vi "Build Project Directory Menu.vi"(9 "Coords":T1, 10 "Project Tree Menu":refnum<k9>, 11 "Project Tree":refnum<vi>) -> (3 "Discard":bool)   [LabVIEW 2015, in "Editor.lvclass"]
uses:
  Editor.lvclass
  <vilib>/Utility/miscctls.llb/LVPoint32TypeDef.ctl
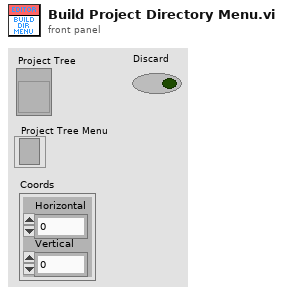
[diagram p1: front panel]
types:
  T1 = typedef "LVPoint32TypeDef.ctl" = cluster{"Horizontal":i32, "Vertical":i32}
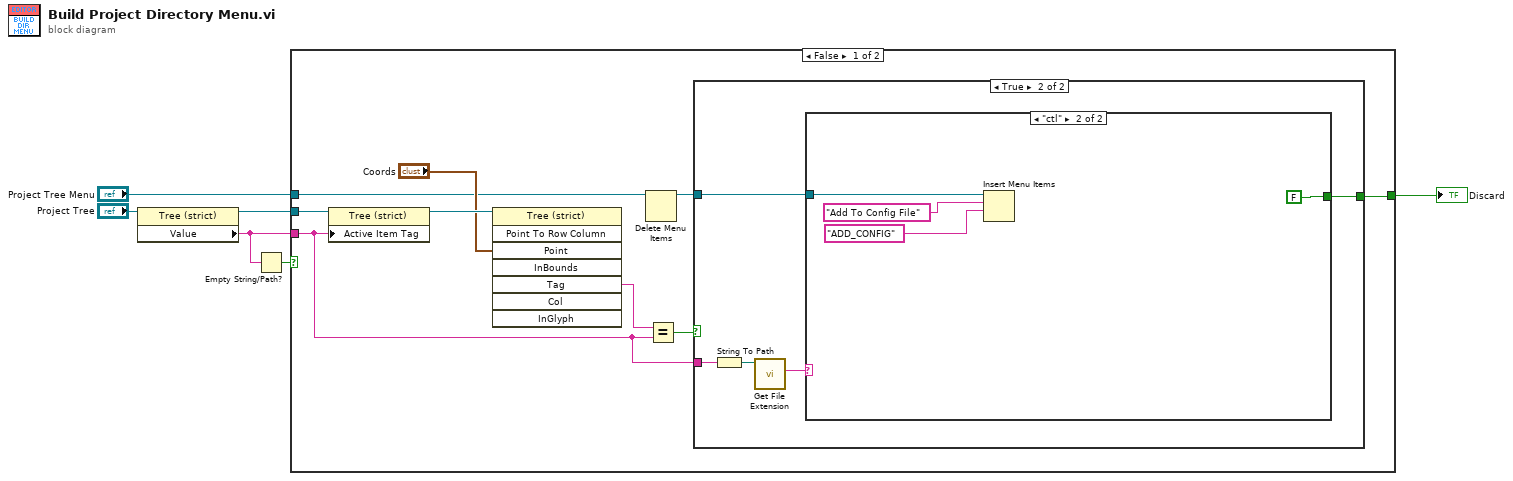
[diagram p0: block diagram]
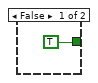
[diagram p2: hidden frame]
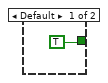
[diagram p3: hidden frame]
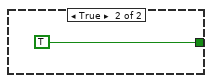
[diagram p4: hidden frame]
diagram:
  n1 = property class="Tree (strict)"(reference="Project Tree") -> (reference out=w6:refnum<vi>, "Value"=w5:string)  [unwired: 1 in, 1 out]
  n2 = Empty String/Path?(string/path=w5) -> (empty?=w4:bool)
  n3 = case shown="False" w4 {
    tunnel: w6 -> [w15 _]
    tunnel: w5 -> [w9 _]
    tunnel: "Project Tree Menu" -> [w11 _]
    tunnel: [w7 TRUE] -> w2
    frame False {
      n4 = property class="Tree (strict)"(reference=w15, "Active Item Tag"=w9) -> (reference out=w14:refnum<vi>)  [unwired: 1 in, 1 out]
      n5 = invoke class="Tree (strict)" method="Point To Row Column"(reference=w14, "Point"="Coords") -> ("Tag"=w12:string)  [unwired: 6 in, 7 out]
      n6 = Delete Menu Items(9:w11) -> (3:w8:refnum<k9>)  [unwired: 3 in, 1 out]
      n7 = Equal?(x=w12, y=w9) -> (x = y?=w10:bool)
      n8 = case shown="True" w10 {
        tunnel: w9 -> [_ w20]
        tunnel: w8 -> [_ w18]
        tunnel: [TRUE w17] -> w7
        frame False {
        }
        frame True {
          n9 = String To Path(string=w20) -> (path=w21:path)
          n10 = call <vilib>:"Get File Extension.vi"("file"=w21) -> ("lowercase file extension"=w19:string)  [unwired: 6 in, 4 out]
          n11 = case shown="\"ctl\"" w19 {
            tunnel: w18 -> [_ w26]
            tunnel: [TRUE FALSE] -> w17
            frame Default {
            }
            frame "ctl" {
              n12 = Insert Menu Items(7:"ADD_CONFIG", 8:"Add To Config File", 9:w26) -> ()  [unwired: 3 in, 3 out]
            }
          }
        }
      }
    }
    frame True {
    }
  }
  "Discard" <- w2
